vi "Write Tx Sim Option.vi"(8 "error in (no error)":errorcluster, 10 "Sim Option":T1, 11 "Node Ptr":T2 format="%.0x") -> (0 "error out":errorcluster, 3 "Node Ptr out":T2 format="%.0x")   [LabVIEW 2019, in "UDP-Custom-Device System Explorer.lvlib" / "Buffered Data Packet.lvlib"]
uses:
  Buffered Data Packet.lvlib
  <vilib>/NI VeriStand/Custom Device API/Custom Device Item Ref.ctl
  Shared/Types/Shared - Transmit Sim Options.ctl
  Shared/Constants.vi
  <vilib>/NI VeriStand/Custom Device API/Set Item Property (U16).vi
  <vilib>/NI VeriStand/Custom Device API/Custom Device API.lvlib
  Shared/UDP-Custom-Device Shared.lvlib
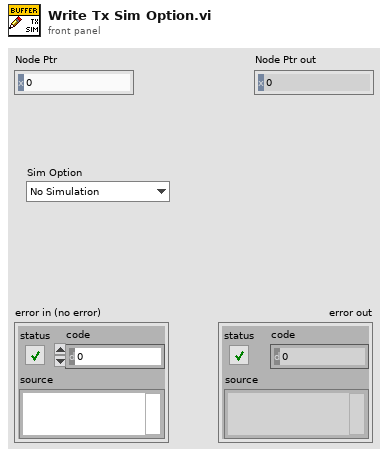
[diagram p1: front panel]
types:
  T1 = typedef "UDP-Custom-Device Shared.lvlib/Shared - Transmit Sim Options.ctl" = enum16{"No Simulation", "Counter", "Full Buffer", "FIFO Test", "FIFO + Port Test"}
  T2 = typedef "Custom Device API.lvlib/Custom Device Item Ref.ctl" = u64
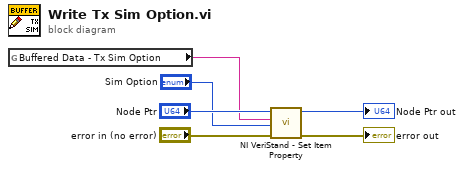
[diagram p0: block diagram]
diagram:
  n1 = global read "Constants.vi" "Buffered Data - Tx Sim Option"() -> (w1:string)
  n2 = call-poly <vilib>:"NI VeriStand - Set Item Property.vi"("error in (no error)"="error in (no error)", "Value"="Sim Option", "Property Name"=w1, "Item Ref in"="Node Ptr") -> ("error out"=→"error out":errorcluster, "Item Ref out"=→"Node Ptr out":T2)  [unwired: 5 in, 1 out]
